vi "To CSV File.vi"(8 "error in (no error)":errorcluster, 9 "Path":path, 10 "engine configuration":refnum<class "engine configuration.lvclass">, 11 "Modbus Module editor node in":refnum<class "Modbus Module editor node.lvclass">) -> (0 "error out":errorcluster, 3 "Modbus Module editor node out":refnum<class "Modbus Module editor node.lvclass">)   [LabVIEW 2015, in "Modbus Module editor node.lvclass"]
uses:
  Modbus Module editor node.lvclass
  <vilib>/NI/Module Execution Interface/Engine Configuration/engine configuration.lvclass
  module/configuration/Modbus Module configuration.lvclass
  <vilib>/NI/Configuration Framework/serializable configuration/NISE_CEF_serializable configuration.lvclass/NISE_CEF_serializable configuration.ctl
  <vilib>/NI/Tag Bus/tag/tag descriptor.lvclass/tag descriptor.ctl
  <vilib>/Utility/LVClass/Get LV Class Name.vi
  <vilib>/NI/Configuration Framework/error generator/NISE_error generator.vi
  <vilib>/NI/Configuration Framework/serializable configuration/NISE_CEF_serializable configuration.lvclass
  <vilib>/NI/Tag Bus/tag/tag descriptor.lvclass
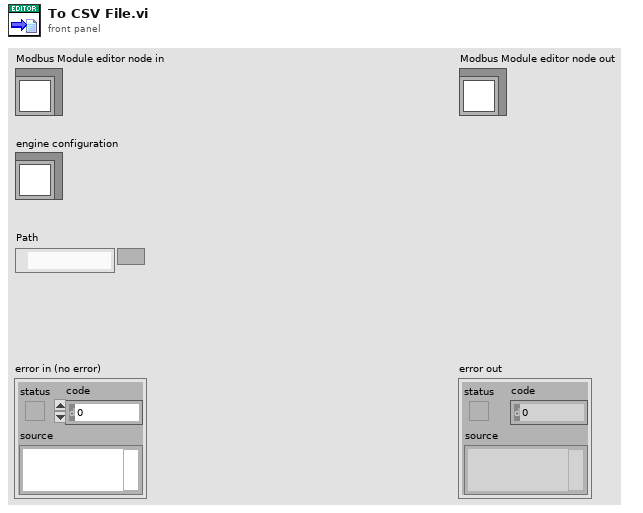
[diagram p1: front panel]
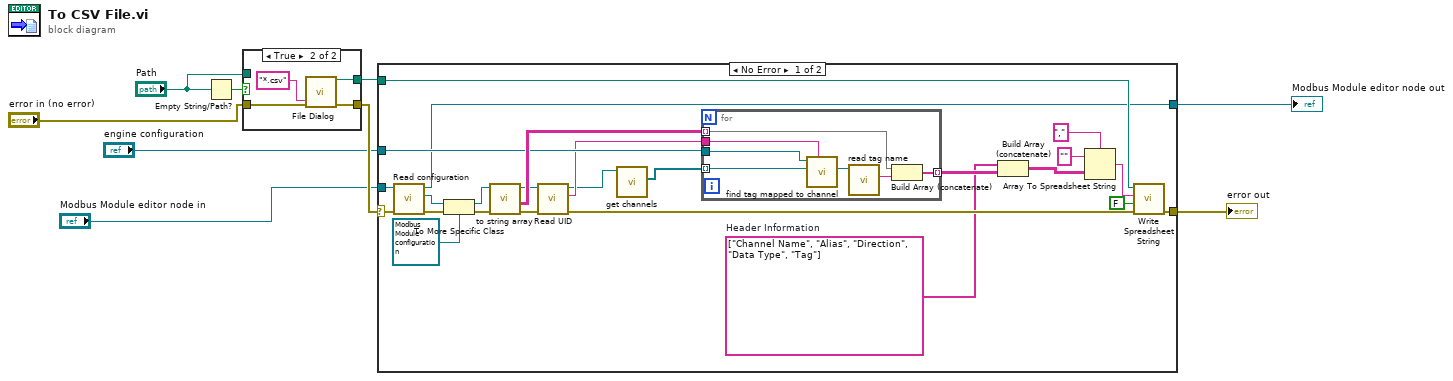
[diagram p0: block diagram]
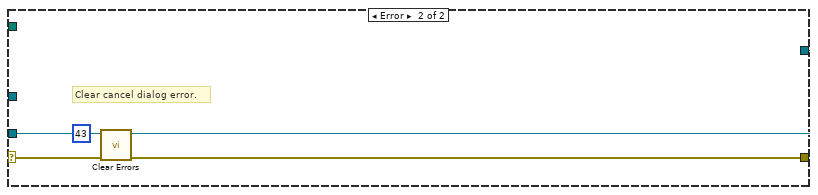
[diagram p3: hidden frame]
diagram:
  n1 = Empty String/Path?(string/path="Path") -> (empty?=w9:bool)
  n2 = case shown="True" w9 {
    tunnel: "error in (no error)" -> [w10 w14]
    tunnel: [w10 w13] -> w7
    tunnel: [w11 w12] -> w8
    tunnel: "Path" -> [w11 _]
    frame False {
    }
    frame True {
      n3 = call "File Dialog"("error in"=w14, "pattern (all files)"="*.csv") -> ("selected path"=w12:path, "error out"=w13:errorcluster)  [unwired: 10 in, 2 out]
    }
  }
  n4 = case shown="No Error" w7 {
    selector: w7 -> [w27 w50]
    tunnel: [w38 w49] -> w2
    tunnel: [w26 w51] -> w3
    tunnel: "Modbus Module editor node in" -> [w28 w51]
    tunnel: w8 -> [w34 _]
    tunnel: "engine configuration" -> [w31 _]
    frame No Error {
      w16 = string[] ["Channel Name", "Alias", "Direction", "Data Type", "Tag"]  # Header Information
      n5 = call-dynamic "Read configuration.vi"("error in"=w27, "Modbus Slave editor node in"=w28) -> ("error out"=w25:errorcluster, "configuration"=w24:refnum<class "NISE_CEF_serializable configuration.lvclass">, "Modbus Slave editor node out"=w26:refnum<class "Modbus Module editor node.lvclass">)  [unwired: 7 in]
      n6 = To More Specific Class(target class=refnum<class "Modbus Module configuration.lvclass"> refnum ("Modbus Module configuration"), reference=w24, error in=w25) -> (specific class reference=w40:refnum<class "Modbus Module configuration.lvclass">, error out=w39:errorcluster)
      n7 = call-dynamic "to string array.vi"("error in (no error)"=w39, "module configuration in"=w40) -> ("error out"=w22:errorcluster, "Array"=w33:string[][], "module configuration out"=w23:refnum<class "Modbus Module configuration.lvclass">)  [unwired: 6 in, 1 out]
      n8 = call <vilib>:"Read UID.vi"("error in"=w22, "configuration in"=w23) -> ("error out"=w20:errorcluster, "instance id"=w30:string, "configuration out"=w19:refnum<class "Modbus Module configuration.lvclass">)  [unwired: 7 in]
      n9 = call-dynamic "get channels.vi"("Modbus Slave configuration in"=w19) -> ("channels"=w18:refnum<class "TBM channel.lvclass">[])  [unwired: 9 in, 1 out]
      n10 = for {
        tunnel: w33 -> [w45] mode=indexing
        tunnel: [w43] -> w32 mode=indexing
        tunnel: w18 -> [w41] mode=indexing
        tunnel: w31 -> [w47]
        tunnel: w30 -> [w42]
        n11 = call <vilib>:"find tag mapped to channel.vi"("owner"=w42, "channel"=w41, "engine configuration in"=w47) -> ("tag"=w46:refnum<class "tag descriptor.lvclass">)  [unwired: 6 in, 2 out]
        n12 = call <vilib>:"read tag name.vi"("system tag in"=w46) -> ("name"=w44:string)  [unwired: 8 in, 2 out]
        n13 = Build Array (concatenate)(w45, w44) -> (w43:string[])
      }
      n14 = Build Array (concatenate)(w16, w32) -> (w17:string[][])
      n15 = Array To Spreadsheet String(delimiter (Tab)=",", array=w17, 3:"" ("format string")) -> (spreadsheet string=w37:string)
      n16 = call <vilib>:"Write Spreadsheet String.vi"("error in"=w20, "append to file? (new file:F)"=FALSE, "spreadsheet string"=w37, "file path (dialog if empty)"=w34) -> ("error out"=w38:errorcluster)  [unwired: 6 in, 1 out]
    }
    frame Error {
      # "Clear cancel dialog error."
      n17 = call <vilib>:"Clear Errors.vi"("error in (no error)"=w50, "specific error code to clear (0: all)"=43) -> ("error out"=w49:errorcluster)  [unwired: 4 in, 1 out]
    }
  }
  "error out" <- w2
  "Modbus Module editor node out" <- w3
